vi "_readNull.vi"(8 "error in (no error)":errorcluster, 11 "tJSONParser in":refnum<class "tJSONParser.lvclass">) -> (0 "error out":errorcluster, 2 "tBSONNull out":refnum<class "tBSONNull.lvclass">, 3 "tJSONParser out":refnum<class "tJSONParser.lvclass">)   [LabVIEW 2013, in "JSON.lvlib" / "tJSONParser.lvclass"]
doc: "Reads a null value form a string : value pair and retruns it as a tBSONElement object for storage in a tBSONDocument object."
uses:
  tJSONParser.lvclass
  BSON/BSONElements/tBSONNull/tBSONNull.lvclass
  _error.ctl
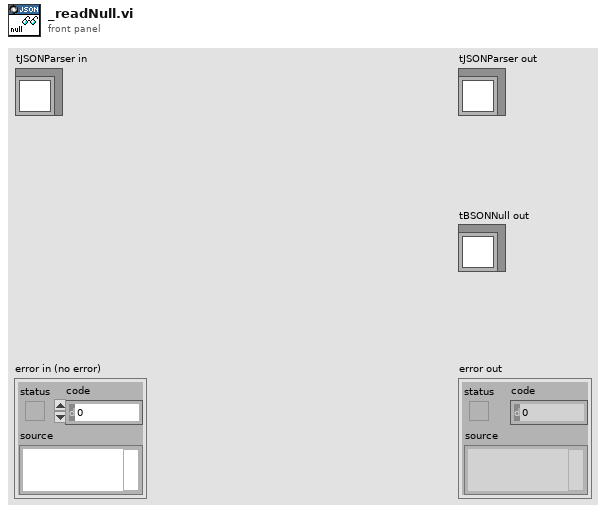
[diagram p1: front panel]
types:
  T1 = typedef "JSON.lvlib/tJSONParser.lvclass/_error.ctl" = enum16{"Missing Object Open", "Missing Pair Separator", "Missing Object End Or Separator", "Missing Pair String", "Unexpected Token", "Missing Array End Or Separator", "Invalid Escape Sequence", "Unexpected End Of File", "Invalid Unicode", "Unexpected End Of Line", "Invalid Numerical Constant"}
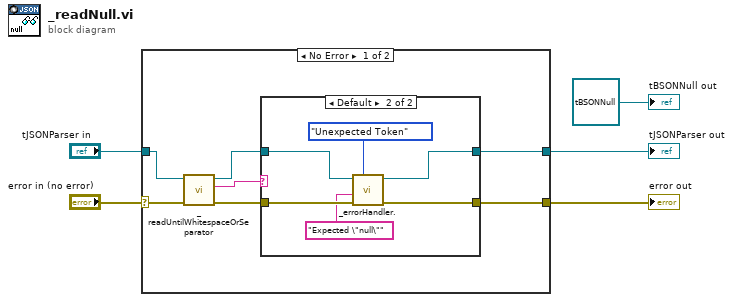
[diagram p0: block diagram]
diagram:
  n1 = case shown="No Error" "error in (no error)" {
    selector: "error in (no error)" -> [w12 w22]
    tunnel: [w8 w22] -> w4
    tunnel: [w10 w21] -> w2
    tunnel: "tJSONParser in" -> [w9 w21]
    frame No Error {
      n2 = call "_readUntilWhitespaceOrSeparator.vi"("error in (no error)"=w12, "tJSONParser in"=w9) -> ("error out"=w6:errorcluster, "String Out"=w7:string, "tJSONParser out"=w11:refnum<class "tJSONParser.lvclass">)  [unwired: 7 in]
      n3 = case shown="Default" w7 {
        tunnel: w6 -> [w13 w20]
        tunnel: w11 -> [w14 w19]
        tunnel: [w14 w16] -> w10
        tunnel: [w13 w15] -> w8
        frame "null" {
        }
        frame Default {
          n4 = call "_errorHandler..vi"("error in (no error)"=w20, "Additional Text"="Expected \"null\"", "Error Type"=_error."Unexpected Token", "JSON Parser In"=w19) -> ("error out"=w15:errorcluster, "JSON Parser Out"=w16:refnum<class "tJSONParser.lvclass">)  [unwired: 6 in]
        }
      }
    }
    frame Error {
    }
  }
  "error out" <- w4
  "tJSONParser out" <- w2
  "tBSONNull out" <- refnum<class "tBSONNull.lvclass"> refnum ("lvMongoDriver.lvlib:BSON.lvlib:tBSONNull.lvclass")
